vi "Build Description String.vi"(8 "error in (no error)":errorcluster, 11 "Image Assertion in":refnum<class "Image Assertion.lvclass">) -> (0 "error out":errorcluster, 1 "Description":string, 2 "Subtype String":string, 3 "Image Assertion out":refnum<class "Image Assertion.lvclass">)   [LabVIEW 2020, in "MacroAssert.lvlib" / "Image Assertion.lvclass"]
doc: "Builds a string to describe what <B>Step</B> does."
uses:
  Image Assertion.lvclass
  C:/Users/acasalen/Documents/LabVIEW Data/Projects/MacroAssert/source/Classes/Assertion Step/Assertion Step.lvclass
  Image Assertion.lvclass/Image Assertion.ctl
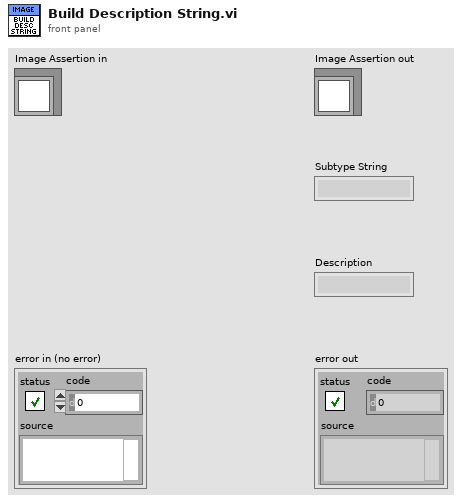
[diagram p1: front panel]
types:
  T1 = typedef "MacroAssert.lvlib/Image Assertion.lvclass/Image Assertion Type.ctl" = enum16{"Control Image", "VI Image", "Window Image", "Cursor Icon"}
  T2 = typedef "MacroAssert.lvlib/Image Assertion.lvclass/Image Comparator.ctl" = enum16{"Is less than or equal to", "Is greater than or equal to"}
  T3 = typedef "MacroAssert.lvlib/Image Assertion.lvclass/Compare Method.ctl" = enum16{"Mean Squared Error", "Peak Signal-to-Noise Ratio"}
  T4 = typedef "MacroAssert.lvlib/Image Assertion.lvclass/Image Units.ctl" = enum16{"Pixels", "Percent"}
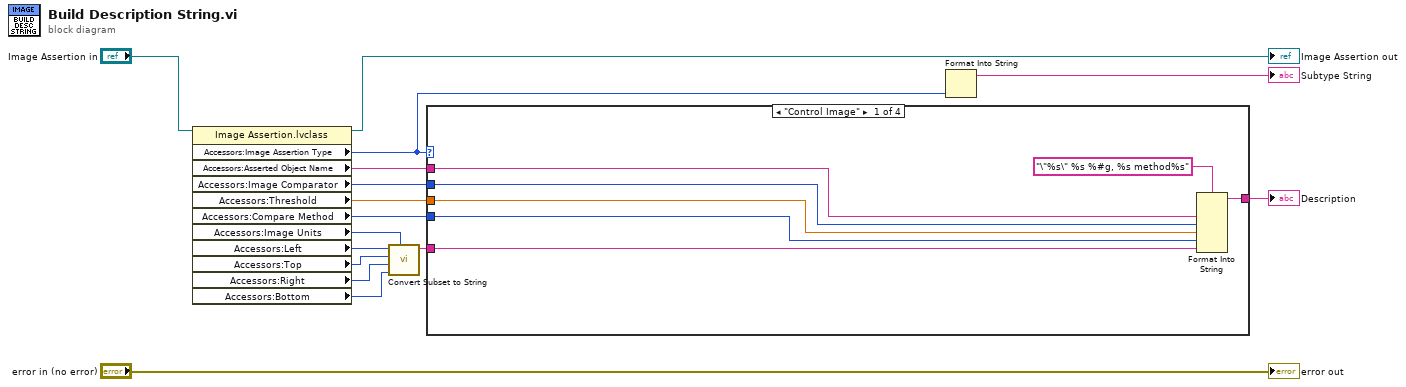
[diagram p0: block diagram]
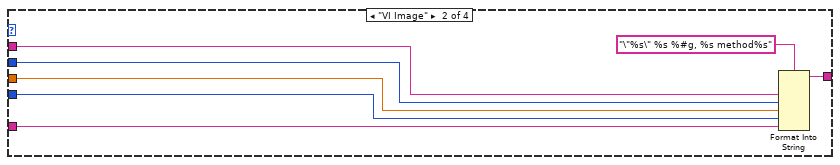
[diagram p2: hidden frame]
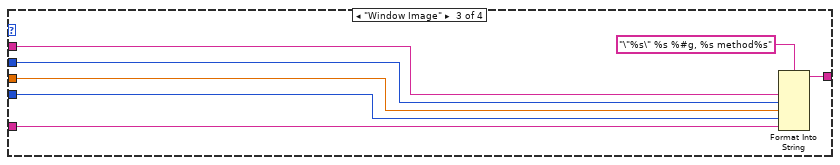
[diagram p3: hidden frame]
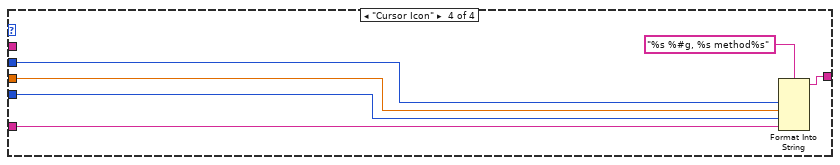
[diagram p4: hidden frame]
diagram:
  n1 = property class="Image Assertion.lvclass"(reference="Image Assertion in") -> (reference out=→"Image Assertion out":refnum<class "Image Assertion.lvclass">, "Accessors:Image Assertion Type"=w7:T1, "Accessors:Asserted Object Name"=w14:string, "Accessors:Image Comparator"=w11:T2, "Accessors:Threshold"=w10:dbl, "Accessors:Compare Method"=w9:T3, "Accessors:Image Units"=w6:T4, "Accessors:Left"=w5:i16, "Accessors:Top"=w4:i16, "Accessors:Right"=w3:i16, "Accessors:Bottom"=w2:i16)  [unwired: 1 in, 1 out]
  n2 = call "Convert Subset to String.vi"("Image Units"=w6, "Bottom"=w2, "Right"=w3, "Top"=w4, "Left"=w5) -> ("Subset String"=w1:string)  [unwired: 6 in]
  n3 = case shown="\"Control Image\"" w7 {
    tunnel: w14 -> [w22 w29 w36 _]
    tunnel: [w21 w28 w35 w42] -> w13
    tunnel: w11 -> [w20 w27 w34 w41]
    tunnel: w10 -> [w19 w26 w33 w40]
    tunnel: w9 -> [w18 w25 w32 w39]
    tunnel: w1 -> [w17 w24 w31 w38]
    frame "Control Image" {
      n4 = Format Into String(format string="\"%s\" %s %#g, %s method%s", w22, w20, w19, w18, w17) -> (resulting string=w21:string)  [unwired: 2 in, 1 out]
    }
    frame "VI Image" {
      n5 = Format Into String(format string="\"%s\" %s %#g, %s method%s", w29, w27, w26, w25, w24) -> (resulting string=w28:string)  [unwired: 2 in, 1 out]
    }
    frame "Window Image" {
      n6 = Format Into String(format string="\"%s\" %s %#g, %s method%s", w36, w34, w33, w32, w31) -> (resulting string=w35:string)  [unwired: 2 in, 1 out]
    }
    frame "Cursor Icon" {
      n7 = Format Into String(format string="%s %#g, %s method%s", w41, w40, w39, w38) -> (resulting string=w42:string)  [unwired: 2 in, 1 out]
    }
  }
  "Description" <- w13
  n8 = Format Into String(w7) -> (resulting string=→"Subtype String":string)  [unwired: 3 in, 1 out]
  "error out" <- "error in (no error)"
